vi "FPGAmain_utan_output.vi"() -> ()   [LabVIEW 2013]
uses:
  FPGA/DataMode.ctl
  FPGA/AcquireState.ctl
  FPGA/Input_5782/5782_states.ctl
  <vilib>/Platform/TimedLoop/XDataNode/timing_clust.ctl
  <vilib>/Platform/TimedLoop/XDataNode/nitl_modes.ctl
  <vilib>/Platform/TimedLoop/XDataNode/wakeup.ctl
  <vilib>/rvi/Emulation/niFpgaSctlEmulationGetInTimedLoop.vi
  <vilib>/rvi/Emulation/niFpgaEmulationReportErrorSimple.vi
  <vilib>/rvi/Emulation/niFpgaGetClockAttributes.vi
  <vilib>/rvi/eio/common/nirviEmuTemplateMethod_errors.vi
  <vilib>/rvi/Emulation/niFpgaCriticalErrorInLSC.vi
  <vilib>/rvi/FIFO/Fifo_Resource/nirvififoEmulationWriteFpgaImpl.vi
  <vilib>/rvi/DataTransferAndStorage/Container/Common/niFpgaContainerGetUniqueNameForEmu.vi
  <vilib>/rvi/FIFO/Fifo_Resource/nirvififoEmulationReadFpgaImpl.vi
  <vilib>/rvi/DataTransferAndStorage/Register/Emulation/niFpgaRegisterEmulationFpgaImpl.vi
  <instcachedir>/0/niFpgaRegisterEmulationFpgaImpl_DCF4BC0110594B98B44A971D60CEEC4D.lvgen/niFpgaRegisterEmulationFpgaImpl_DCF4BC0110594B98B44A971D60CEEC4D_016.vi
  <instcachedir>/0/niFpgaRegisterEmulationFpgaImpl_DCF4BC0110594B98B44A971D60CEEC4D.lvgen/niFpgaRegisterEmulationFpgaImpl_DCF4BC0110594B98B44A971D60CEEC4D_003.vi
  <instcachedir>/0/niFpgaRegisterEmulationFpgaImpl_DCF4BC0110594B98B44A971D60CEEC4D.lvgen/niFpgaRegisterEmulationFpgaImpl_DCF4BC0110594B98B44A971D60CEEC4D_014.vi
  <instcachedir>/0/niFpgaRegisterEmulationFpgaImpl_DCF4BC0110594B98B44A971D60CEEC4D.lvgen/niFpgaRegisterEmulationFpgaImpl_DCF4BC0110594B98B44A971D60CEEC4D_015.vi
  <vilib>/rvi/interface/RandomDataEmulation/nirviRandomDataMultiElementFPGAFIFO.vi
  <instcachedir>/0/nirviRandomDataMultiElementFPGAFIFO_F2B80EDE0D7944A08478D8D26097D4DB.lvgen/nirviRandomDataMultiElementFPGAFIFO_F2B80EDE0D7944A08478D8D26097D4DB_005.vi
  <vilib>/rvi/interface/RandomDataEmulation/niFpgaRandomDataHandleErrors.vi
  <vilib>/rvi/interface/RandomDataEmulation/nirviRandomDataFPGAFIFO.vi
  <instcachedir>/0/niFpgaRegisterEmulationFpgaImpl_DCF4BC0110594B98B44A971D60CEEC4D.lvgen/niFpgaRegisterEmulationFpgaImpl_DCF4BC0110594B98B44A971D60CEEC4D_009.vi
  <instcachedir>/0/niFpgaRegisterEmulationFpgaImpl_DCF4BC0110594B98B44A971D60CEEC4D.lvgen/niFpgaRegisterEmulationFpgaImpl_DCF4BC0110594B98B44A971D60CEEC4D_013.vi
  <vilib>/Platform/TimedLoop/XDataNode/XDataNode.xnode
  <vilib>/eio/EIONode/EIONode.xnode
  <vilib>/rvi/DataTransferAndStorage/Container/XNode/niFpgaContainer.xnode
  <vilib>/rvi/FIFO/Fifo_Resource/nirvififoEmulationWrite.vi
  <vilib>/rvi/FIFO/Fifo_Resource/nirvififoEmulationRead.vi
  <vilib>/rvi/DataTransferAndStorage/Register/Emulation/niFpgaRegisterEmulation.vi
  <vilib>/rvi/interface/RandomDataEmulation/nirviRandomDataFpgaMultiElementTemplate.vi
  <vilib>/rvi/interface/RandomDataEmulation/nirviRandomDataFpgaReadWriteTemplate.vi
  <vilib>/rvi/FIFO/Fifo_Resource/nirvififoEmulationP2P.vi
  <vilib>/Platform/TimedLoop/XDataNode/XDNodeRunTimeDep.lvlib
  <instrlib>/FlexRIO/Libraries/Helper VIs/NI FlexRIO Helper VIs.lvlib
panel:
  in  "delay phase":fxp<+,64,64>
  in  "AM phase":fxp<+,64,64>
  in  "Phase 5782":fxp<+,64,64>[](array[numeric])=[0.0, 0.0]
  in  "User Command Commit":bool
  in  "User Command":u8
  out "User Command Idle":bool
  out "User Command Status":u8
  in  "User Data 0":u8
  in  "User Data 1":u8
  out "PLL Locked":bool
  out "User Error":bool
  out "Configured?":bool
  in  "FIR coeffs":fxp<+/-,18,18>[](array[numeric])
  in  "Phase output":fxp<+,64,64>[](array[numeric])=[0.0, 0.0, 0.0, 0.0]
  in  "5782 record length":u16=4000 caption="Samples Per Trigger" min=1 step=1
  in  "Trigger Acquisition":bool
  in  "Continuous":bool
  out "IO Module\\Trigger Input":bool
  in  "Mode":T1
  in  "Simulated phase 5782":fxp<+,64,64>[](array[numeric])=[0.0, 0.0]
  in  "Acquisition running":bool
  in  "Samples Per Trigger":i32 min=1 step=1
  in  "Trigger simulated data":bool
  in  "simulated phase 5160":fxp<+,64,64>
  in  "phase 5160":fxp<+,64,64>
  # "Dynamic filter"
  # "Dynamic downsample"
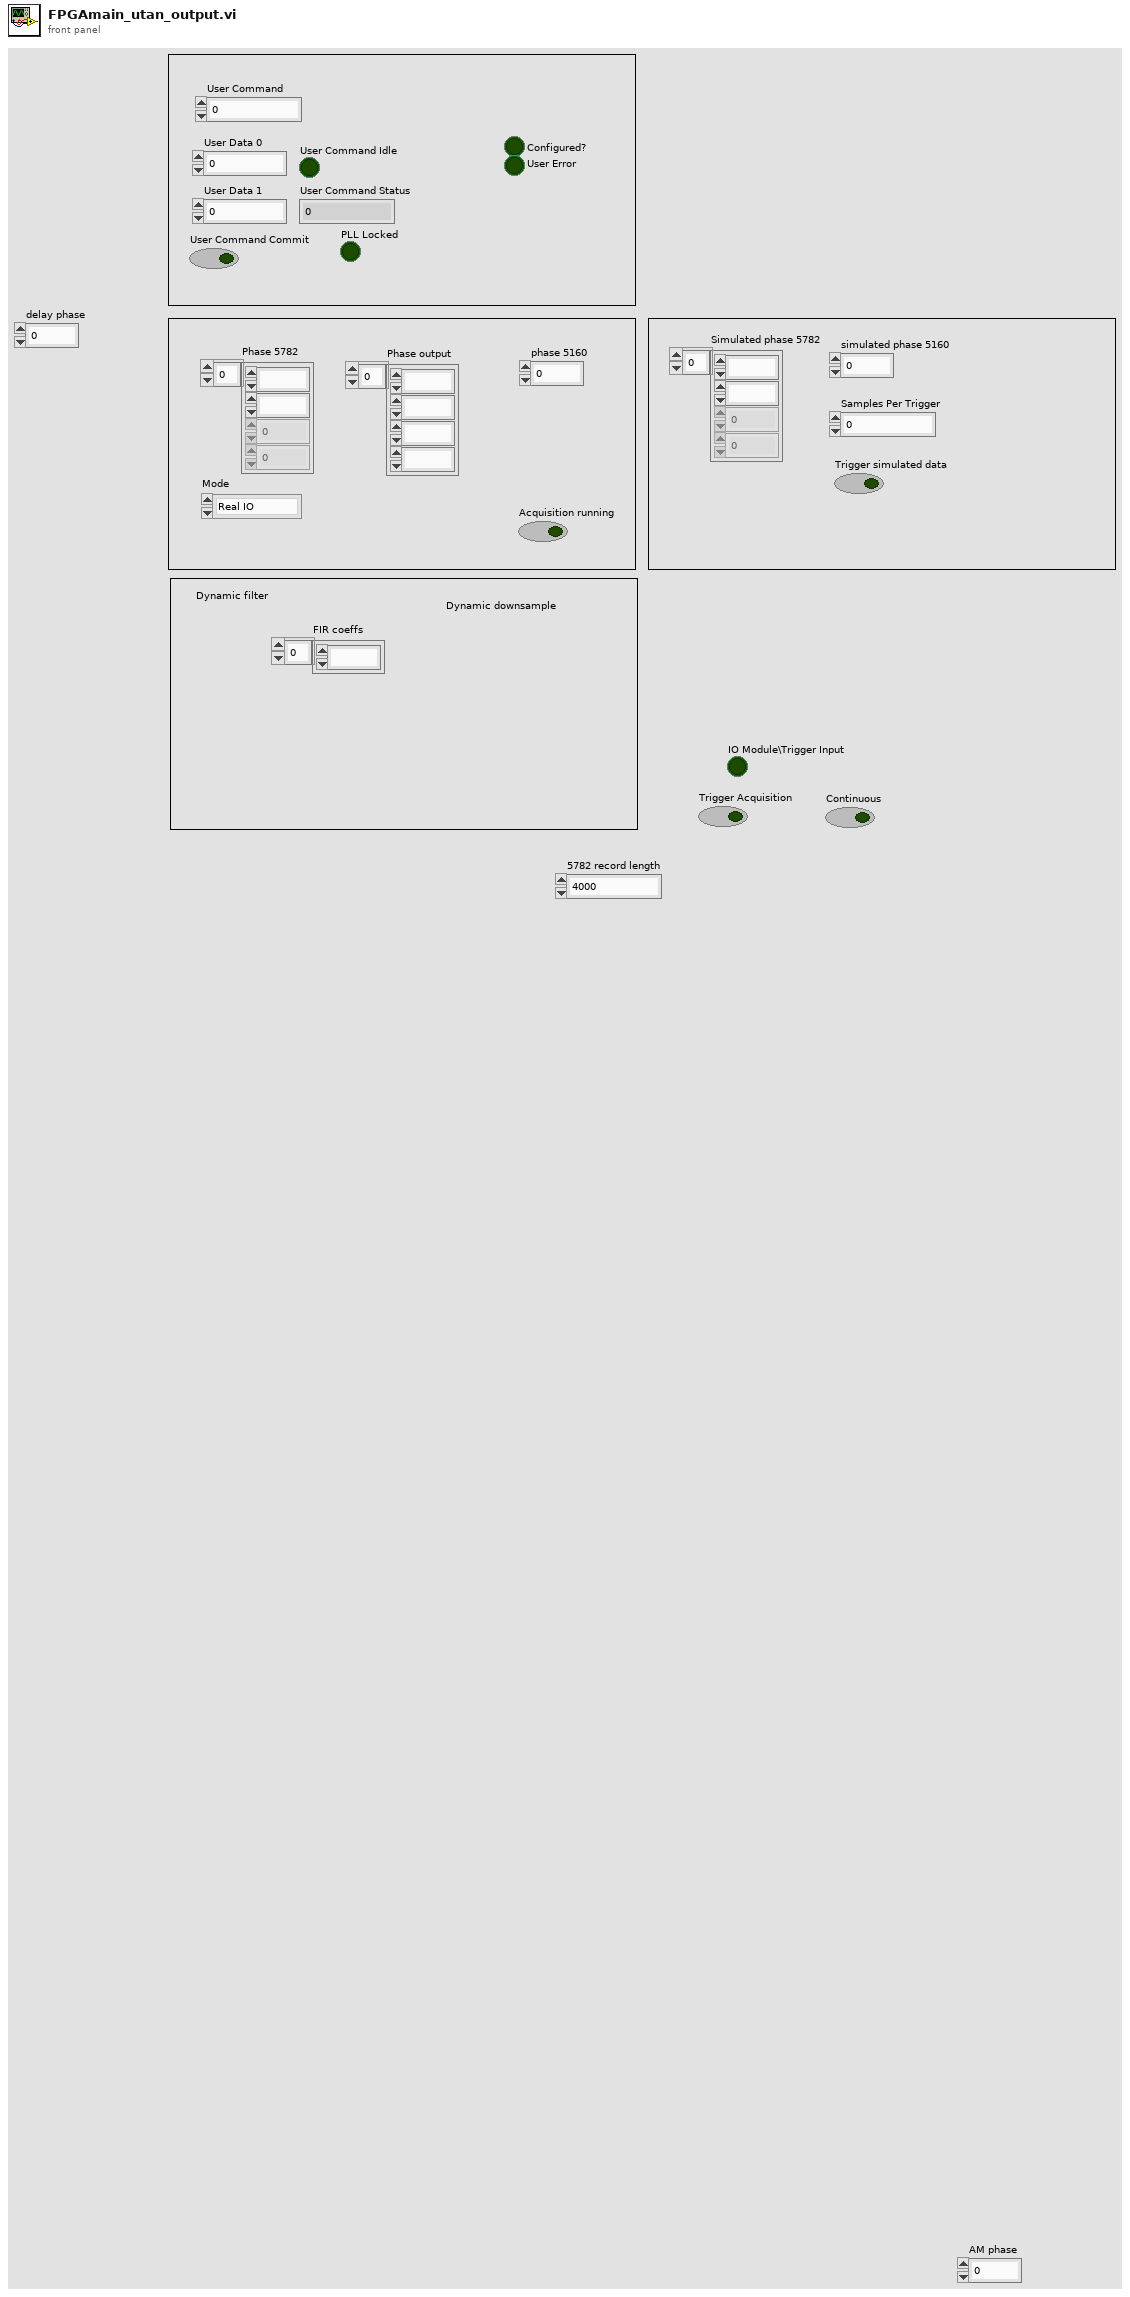
[diagram p1: front panel]
types:
  T1 = typedef "DataMode.ctl" = enum16{"Real IO", "Simulated"}
  T2 = typedef "5782_states.ctl" = enum8{"Wait for trigger", "Acquisition", "Send record length", "Quiet period"}
  T3 = typedef "AcquireState.ctl" = enum8{"Idle", "Acquire"}
  T4 = typedef "XDNodeRunTimeDep.lvlib/timing_clust.ctl" = cluster{"Expected End [f-1]":u64, "Actual End [f-1]":u64, "Finished Late? [f-1]":bool, "Expected End [i-1]":u64, "Actual End [i-1]":u64, "Finished Late? [i-1]":bool, "Expected Start [i]":u64, "Actual Start [i]":u64, "Expected Start [f]":u64, "Actual Start [f]":u64, "Source Name":string, "Structure Name":string, "Period":i64, "Deadline":i64, "Offset":i64, "Start":i64, "Priority":i32, "Timeout":i32, "Mode":T5, "Wakeup Reason":T6, "Error":errorcluster, "Source Type":string, "Secondary Source Type":string, "Global End Time":u64, "Global Start Time":u64, "Frame Duration":u64, "Iteration Duration":u64, "Assigned CPU":i32, "I/O Scan Engine Mode":u32}
  T5 = typedef "XDNodeRunTimeDep.lvlib/nitl_modes.ctl" = enum32{"No Change", "Process missed periods, maintain original phase", "Discard missed periods, maintain original phase", "Process missed periods, ignore original phase", "Discard missed periods, ignore original phase"}
  T6 = typedef "XDNodeRunTimeDep.lvlib/wakeup.ctl" = enum32{"Normal", "Aborted", "Asynchronous wakeup", "Timing source error", "Timed loop error", "Timeout"}
  T7 = typedef "I16 array size 2.ctl" = i16[]
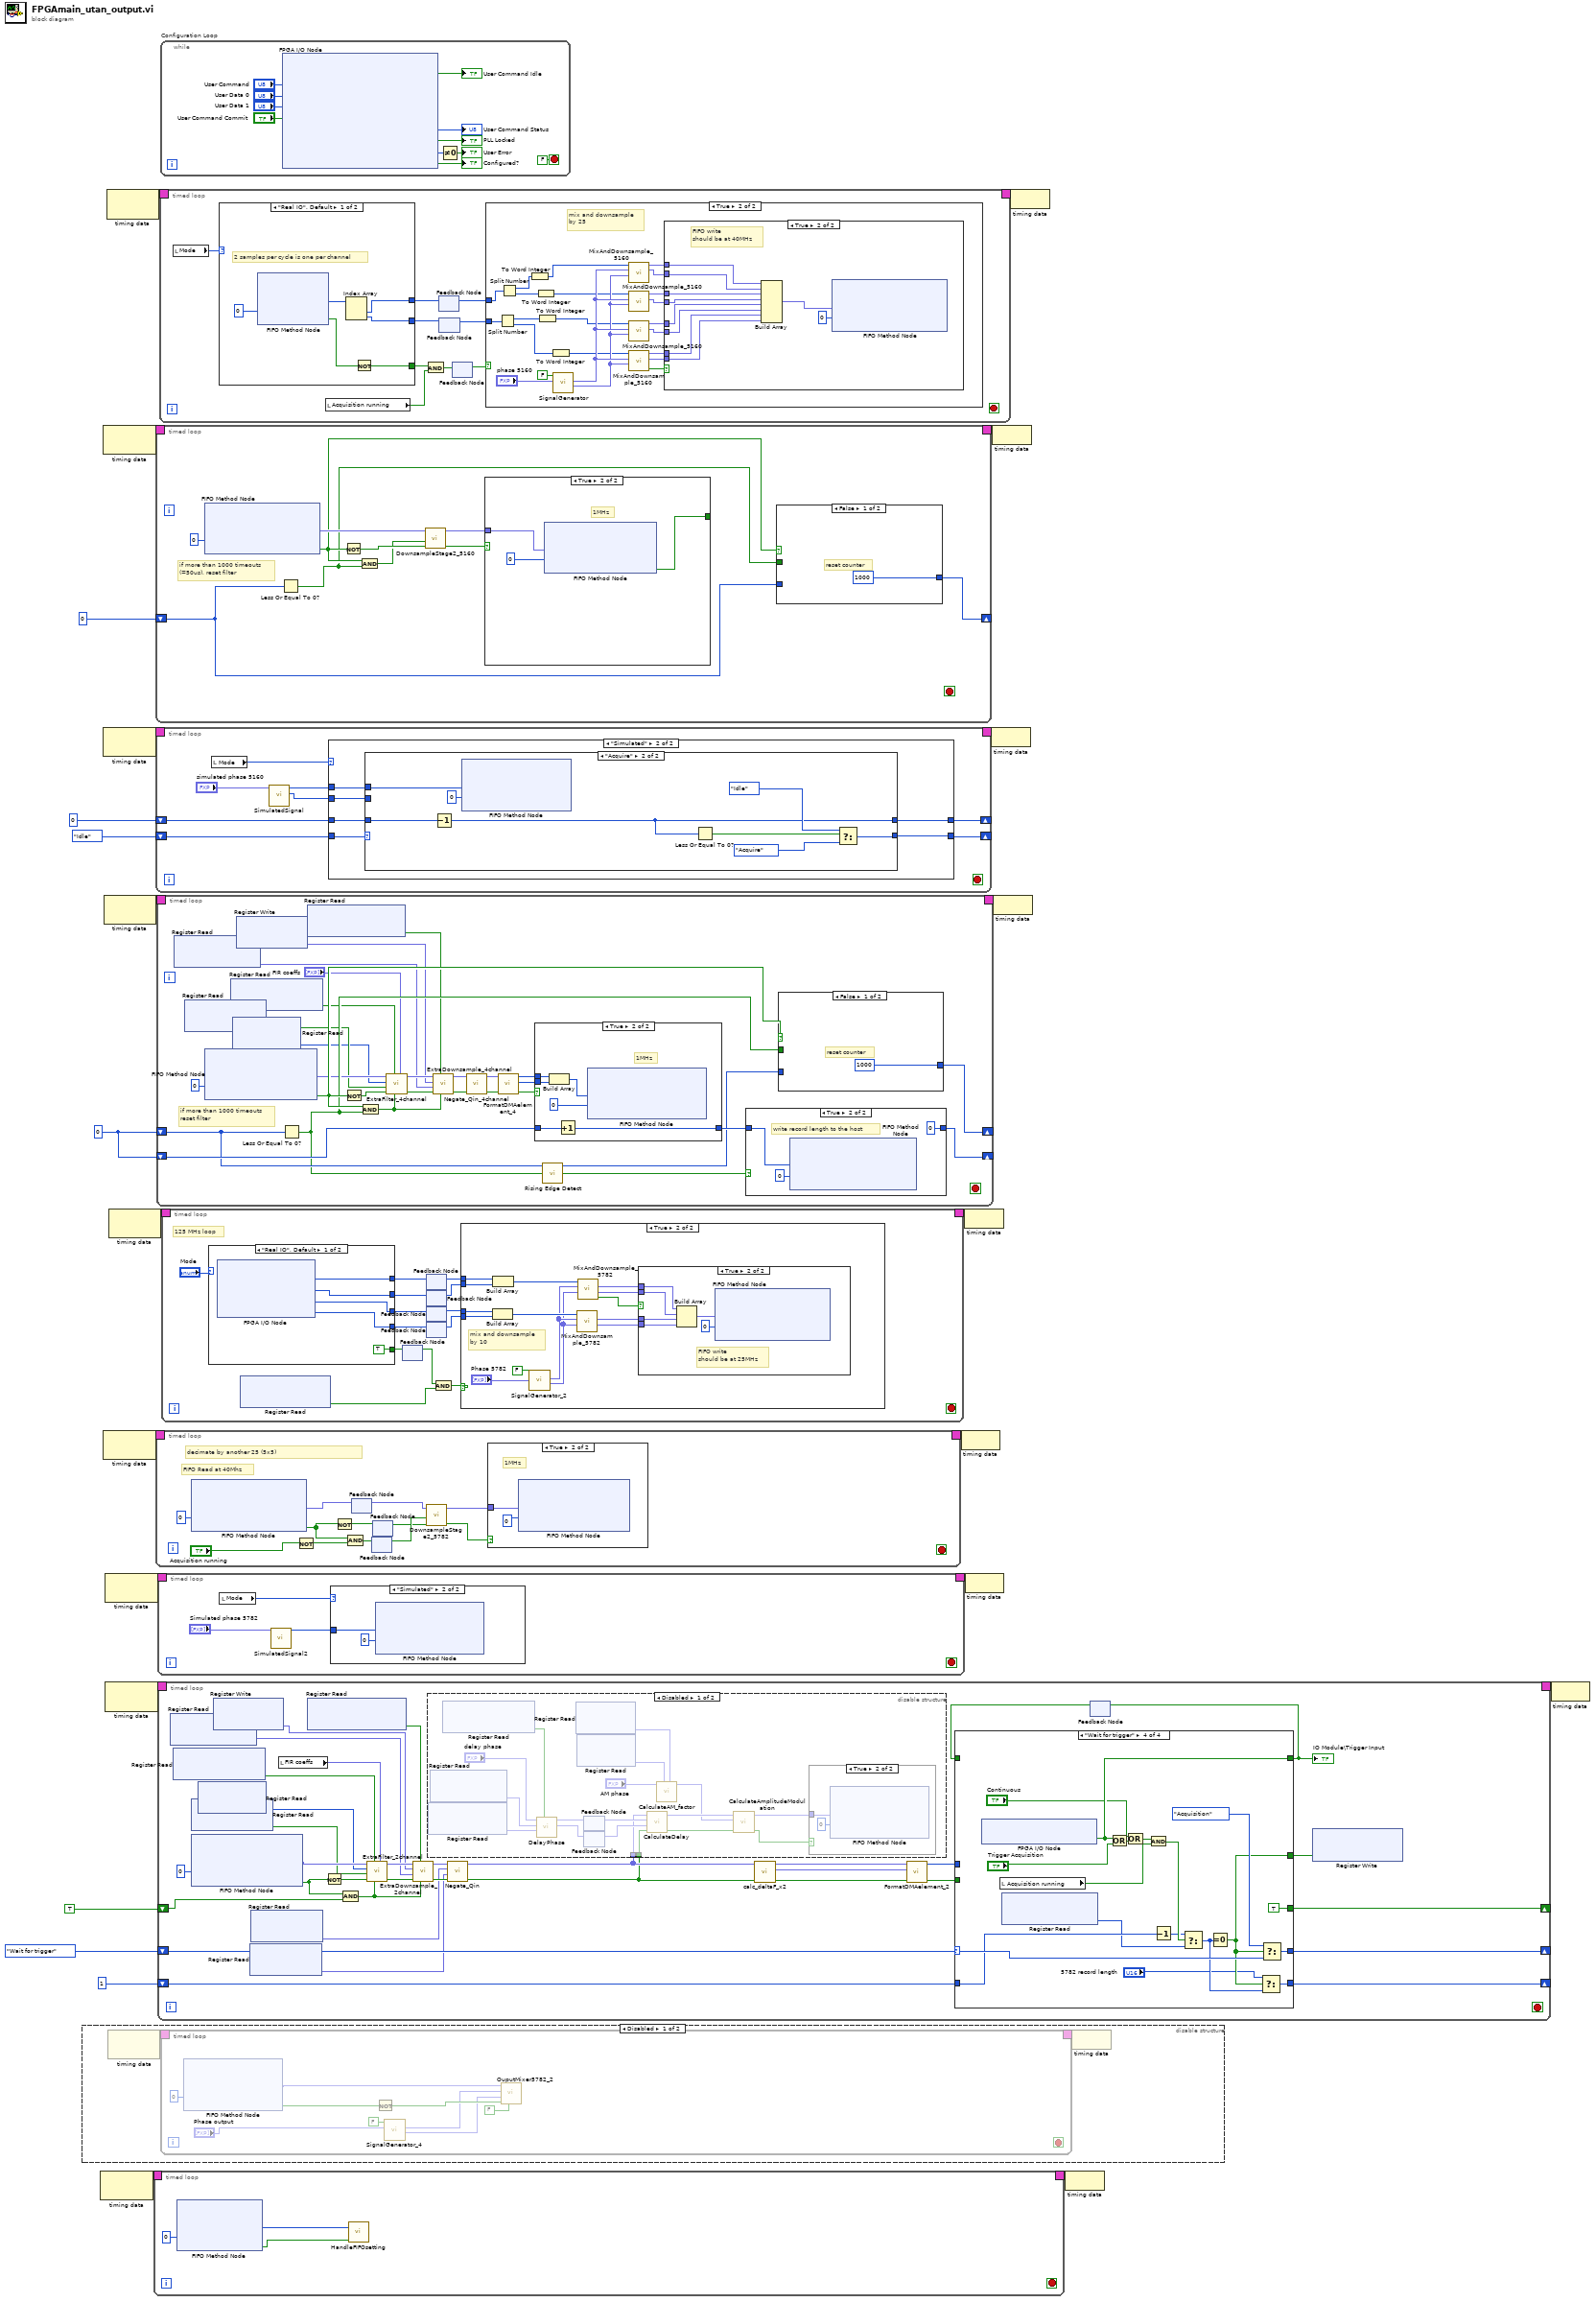
[diagram p0: block diagram]
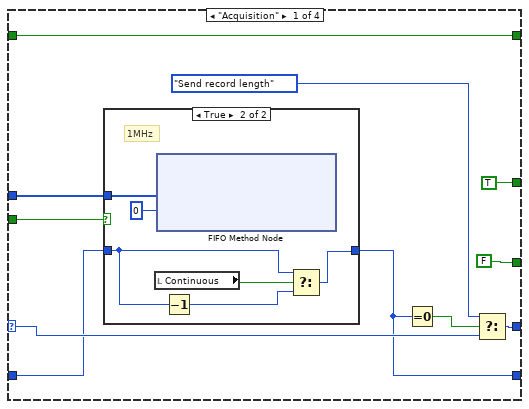
[diagram p5: hidden frame]
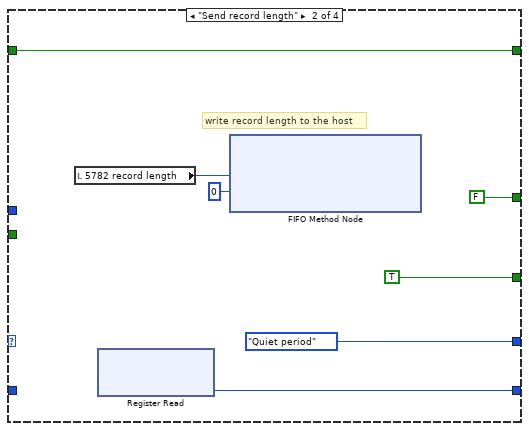
[diagram p7: hidden frame]
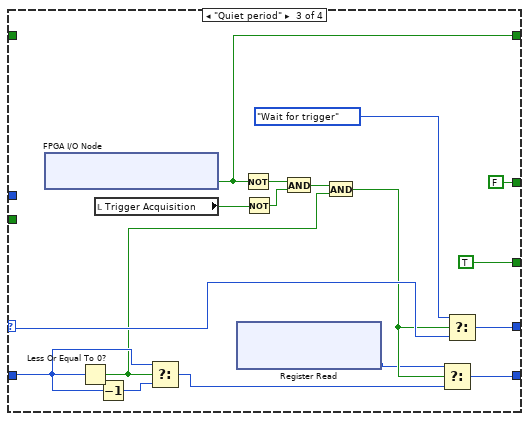
[diagram p8: hidden frame]
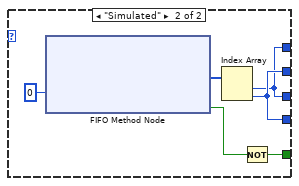
[diagram p11: hidden frame]
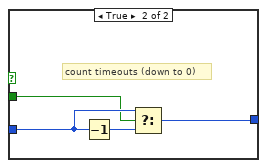
[diagram p14: hidden frame]
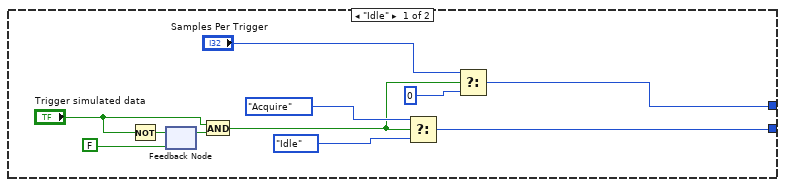
[diagram p18: hidden frame]
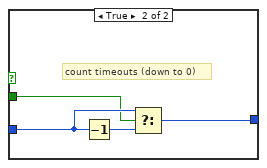
[diagram p19: hidden frame]
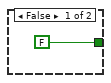
[diagram p20: hidden frame]
diagram:
  w14 = 0 ("y")
  n1 = disable-structure shown="Disabled" {
    frame Disabled {
      n2 = node-c288() -> (w27:T4)  [unwired: 1 in]
      n3 = timed-loop {
        timing: w27 -> [_]
        timing-out: [_] -> w26
        stop <- _ stop-if-true
        n4 = xnode ("FIFO Method Node")("Timeout"=0) -> ("Element"=w28:fxp<+/-,16,14>[], "Timed Out?"=w30:bool)  [unwired: 1 in, 1 out]
        n5 = Not(x=w30) -> (.not. x?=w34:bool)
        n6 = call "SignalGenerator_4.vi"("Phase"="Phase output", "reset"=FALSE) -> ("Sine out"=w31:fxp<+/-,16,0>[], "Cosine out"=w32:fxp<+/-,16,0>[])  [unwired: 8 in]
        n7 = call "OuputMixer5782_2.vi"("reset"=FALSE, "valid in"=w34, "Sine in"=w31, "Cosine in"=w32, "Data in"=w28) -> ()  [unwired: 5 in, 2 out]
      }
      n8 = node-c288(w26) -> ()
    }
    frame Enabled {
    }
  }
  n9 = node-c288() -> (w5:T4)  [unwired: 1 in]
  n10 = node-c288() -> (w23:T4)  [unwired: 1 in]
  n11 = node-c288() -> (w21:T4)  [unwired: 1 in]
  n12 = node-c288() -> (w11:T4)  [unwired: 1 in]
  n13 = node-c288() -> (w16:T4)  [unwired: 1 in]
  n14 = node-c288() -> (w13:T4)  [unwired: 1 in]
  n15 = node-c288() -> (w7:T4)  [unwired: 1 in]
  n16 = node-c288() -> (w25:T4)  [unwired: 1 in]
  n17 = node-c288() -> (w9:T4)  [unwired: 1 in]
  n18 = timed-loop {
    timing: w5 -> [_]
    timing-out: [_] -> w4
    stop <- _ stop-if-true
    n19 = xnode ("FIFO Method Node")("Timeout"=0) -> ("Element"=w42:u64, "Timed Out?"=w41:bool)  [unwired: 1 in, 1 out]
    n20 = call "HandleFIFOsetting.vi"("timed out"=w41, "Value"=w42) -> ()  [unwired: 10 in]
  }
  n21 = timed-loop {
    timing: w23 -> [_]
    timing-out: [_] -> w22
    shift-right: [w48] -> _
    shift-left: 0 ("y") -> [w47]
    stop <- _ stop-if-true
    # "if more than 1000 timeouts\n(=50us), reset filter"
    n22 = xnode ("FIFO Method Node")("Timeout"=0) -> ("Element"=w52:fxp<+/-,16,14>[], "Timed Out?"=w49:bool)  [unwired: 1 in, 1 out]
    n23 = Less Or Equal To 0?(x=w47) -> (x <= 0?=w46:bool)
    n24 = Not(x=w49) -> (.not. x?=w53:bool)
    n25 = And(x=w49, y=w46) -> (x .and. y?=w50:bool)
    n26 = call "DownsampleStage2_5160.vi"("valid in"=w53, "reset"=w50, "Element"=w52) -> ("valid out"=w54:bool, "Array"=w55:fxp<+/-,16,14>[])  [unwired: 7 in]
    n27 = case shown="True" w54 {
      tunnel: w55 -> [_ w62]
      tunnel: [FALSE ("Timed Out?") w63] -> _
      frame False {
      }
      frame True {
        # "1MHz"
        n28 = xnode ("FIFO Method Node")("Element"=w62, "Timeout"=0) -> ("Timed Out?"=w63:bool)  [unwired: 1 in, 1 out]
      }
    }
    n29 = case shown="False" w49 {
      tunnel: w46 -> [_ w58]
      tunnel: w47 -> [_ w59]
      tunnel: [1000 ("y") w57] -> w48
      frame False {
        # "reset counter"
      }
      frame True {
        # "count timeouts (down to 0)"
        n30 = Decrement(x=w59) -> (x-1=w60:i32)
        n31 = Select(t=w59, s=w58, f=w60) -> (s? t:f=w57:i32)
      }
    }
  }
  n32 = timed-loop {
    timing: w21 -> [_]
    timing-out: [_] -> w20
    shift-right: [w70] -> _
    shift-left: 0 ("f") -> [w69]
    shift-right: [w68] -> _
    shift-left: AcquireState."Idle" ("Acquire State") -> [w67]
    stop <- _ stop-if-true
    n33 = local read "Mode"() -> (w74:T1)
    n34 = call "SimulatedSignal.vi"("phase"="simulated phase 5160") -> ("cos output"=w72:i16, "Sample output"=w73:i16)  [unwired: 9 in]
    n35 = case shown="\"Simulated\"" w74 {
      tunnel: w73 -> [_ w82]
      tunnel: w72 -> [_ w77]
      tunnel: [w76 w81] -> w70
      tunnel: w69 -> [w76 w80]
      tunnel: [w75 w79] -> w68
      tunnel: w67 -> [w75 w78]
      frame "Real IO" {
      }
      frame "Simulated" {
        n36 = case shown="\"Acquire\"" w78 {
          tunnel: w80 -> [_ w98]
          tunnel: [w87 w97] -> w79
          tunnel: [w84 w96] -> w81
          tunnel: w82 -> [_ w95]
          tunnel: w77 -> [_ _]
          frame "Idle" {
            n37 = Not(x="Trigger simulated data") -> (.not. x?=w88:bool)
            n38 = feedback #1(FALSE) -> (w89:bool)
            n39 = feedback-in #1(w88) -> ()
            n40 = And(x="Trigger simulated data", y=w89) -> (x .and. y?=w83:bool)
            n41 = Select(t=AcquireState."Acquire" ("Acquire State"), s=w83, f=AcquireState."Idle" ("Acquire State")) -> (s? t:f=w87:T3)
            n42 = Select(t="Samples Per Trigger", s=w83, f=0) -> (s? t:f=w84:i32)
          }
          frame "Acquire" {
            n43 = Decrement(x=w98) -> (x-1=w96:i32)
            n44 = xnode ("FIFO Method Node")("Element"=w95, "Timeout"=0) -> ()  [unwired: 1 in, 2 out]
            n45 = Less Or Equal To 0?(x=w96) -> (x <= 0?=w100:bool)
            n46 = Select(t=AcquireState."Idle" ("Acquire State"), s=w100, f=AcquireState."Acquire" ("Acquire State")) -> (s? t:f=w97:T3)
          }
        }
      }
    }
  }
  n47 = timed-loop {
    timing: w11 -> [_]
    timing-out: [_] -> w10
    stop <- _ stop-if-true
    # "FIFO Read at 40Mhz"
    # "decimate by another 25 (5x5)"
    n48 = xnode ("FIFO Method Node")("Timeout"=0) -> ("Element"=w110:fxp<+/-,16,14>[], "Timed Out?"=w111:bool)  [unwired: 1 in, 1 out]
    n49 = Not(x="Acquisition running") -> (.not. x?=w112:bool)
    n50 = Not(x=w111) -> (.not. x?=w106:bool)
    n51 = And(x=w111, y=w112) -> (x .and. y?=w108:bool)
    n52 = feedback #2() -> (w109:fxp<+/-,16,14>[])  [unwired: 1 in]
    n53 = feedback-in #2(w110) -> ()
    n54 = feedback #3() -> (w107:bool)  [unwired: 1 in]
    n55 = feedback-in #3(w108) -> ()
    n56 = feedback #4() -> (w105:bool)  [unwired: 1 in]
    n57 = feedback-in #4(w106) -> ()
    n58 = call "DownsampleStage2_5782.vi"("valid in"=w105, "reset"=w107, "Data in"=w109) -> ("valid out"=w113:bool, "data out"=w114:fxp<+/-,16,14>[])  [unwired: 7 in]
    n59 = case shown="True" w113 {
      tunnel: w114 -> [_ w116]
      frame False {
      }
      frame True {
        # "1MHz"
        n60 = xnode ("FIFO Method Node")("Element"=w116, "Timeout"=0) -> ()  [unwired: 1 in, 2 out]
      }
    }
  }
  n61 = timed-loop {
    timing: w16 -> [_]
    timing-out: [_] -> w15
    shift-right: [w142] -> _
    shift-left: w14 -> [w141]
    shift-right: [w144] -> _
    shift-left: w14 -> [w146]
    stop <- _ stop-if-true
    # "if more than 1000 timeouts\nreset filter"
    n62 = xnode ("Register Read")() -> ("Data"=w123:fxp<+,8,8>)  [unwired: 1 in, 1 out]
    n63 = xnode ("Register Read")() -> ("Data"=w121:bool)  [unwired: 1 in, 1 out]
    n64 = xnode ("FIFO Method Node")("Timeout"=0) -> ("Element"=w137:fxp<+/-,16,14>[], "Timed Out?"=w143:bool)  [unwired: 1 in, 1 out]
    n65 = xnode ("Register Read")() -> ("Data"=w122:bool)  [unwired: 1 in, 1 out]
    n66 = xnode ("Register Read")() -> ("Data"=w120:i32)  [unwired: 1 in, 1 out]
    n67 = xnode ("Register Write")() -> ("Data"=w124:fxp<+/-,32,1>)  [unwired: 1 in, 1 out]
    n68 = Less Or Equal To 0?(x=w141) -> (x <= 0?=w140:bool)
    n69 = xnode ("Register Read")() -> ("Data"=w125:bool)  [unwired: 1 in, 1 out]
    n70 = Not(x=w143) -> (.not. x?=w136:bool)
    n71 = And(x=w143, y=w140) -> (x .and. y?=w138:bool)
    n72 = call "ExtraFilter_4channel.vi"(5:"new coeffs"="FIR coeffs", "reset"=w138, 7:"new coeffs"=w122, "valid in"=w136, "enable filter"=w121, "new shift"=w120, "Data in"=w137) -> ("valid out"=w127:bool, "Data out"=w128:fxp<+/-,16,14>[])  [unwired: 3 in]
    n73 = call "ExtraDownsample_4channel.vi"("reset"=w138, "Set downsample"=w125, "valid in"=w127, "Downsample"=w123, "CIC Gain"=w124, "Data in"=w128) -> ("valid out"=w129:bool, "Data out"=w132:fxp<+/-,16,14>[])  [unwired: 4 in]
    n74 = call "Negate_Qin_4channel.vi"("valid in"=w129, "Data in"=w132) -> ("valid out"=w130:bool, "Data out"=w131:fxp<+/-,16,14>[])  [unwired: 8 in]
    n75 = call "FormatDMAelement_4.vi"("valid in"=w130, "Data in"=w131) -> ("valid out"=w133:bool, "Element2"=w134:u64, "Element1"=w135:u64)  [unwired: 7 in]
    n76 = case shown="True" w133 {
      tunnel: w135 -> [_ w162]
      tunnel: w134 -> [_ w161]
      tunnel: w146 -> [w157 w159]
      tunnel: [w157 w158] -> w145
      frame False {
      }
      frame True {
        # "1MHz"
        n77 = Build Array(w162, w161) -> (w160:u64[])
        n78 = Increment(x=w159) -> (x+1=w158:i32)
        n79 = xnode ("FIFO Method Node")("Element"=w160, "Timeout"=0) -> ()  [unwired: 1 in, 2 out]
      }
    }
    n80 = call <instrlib>:"Rising Edge Detect.vi"("signal"=w140) -> ("edge detected"=w139:bool)  [unwired: 14 in]
    n81 = case shown="True" w139 {
      tunnel: w145 -> [w153 w154]
      tunnel: [w153 0 ("y")] -> w144
      frame False {
      }
      frame True {
        # "write record length to the host"
        n82 = xnode ("FIFO Method Node")("Element"=w154, "Timeout"=0) -> ()  [unwired: 1 in, 2 out]
      }
    }
    n83 = case shown="False" w143 {
      tunnel: w140 -> [_ w150]
      tunnel: w141 -> [_ w151]
      tunnel: [1000 ("y") w149] -> w142
      frame False {
        # "reset counter"
      }
      frame True {
        # "count timeouts (down to 0)"
        n84 = Decrement(x=w151) -> (x-1=w152:i32)
        n85 = Select(t=w151, s=w150, f=w152) -> (s? t:f=w149:i32)
      }
    }
  }
  n86 = timed-loop {
    timing: w13 -> [_]
    timing-out: [_] -> w12
    stop <- _ stop-if-true
    n87 = local read "Mode"() -> (w168:T1)
    n88 = call "SimulatedSignal2.vi"("Phase"="Simulated phase 5782") -> ("output"=w167:T7)  [unwired: 9 in, 1 out]
    n89 = case shown="\"Simulated\"" w168 {
      tunnel: w167 -> [_ w169]
      frame "Real IO", Default {
      }
      frame "Simulated" {
        n90 = xnode ("FIFO Method Node")("Element"=w169, "Timeout"=0) -> ()  [unwired: 1 in, 2 out]
      }
    }
  }
  n91 = timed-loop {
    timing: w7 -> [_]
    timing-out: [_] -> w6
    shift-right: [w204] -> _
    shift-left: 5782_states."Wait for trigger" ("5782 states") -> [w206]
    shift-right: [w203] -> _
    shift-left: u16 1 ("trigger samples") -> [w205]
    shift-right: [w192] -> _
    shift-left: TRUE -> [w195]
    stop <- _ stop-if-true
    n92 = xnode ("Register Read")() -> ("Data"=w177:fxp<+,8,8>)  [unwired: 1 in, 1 out]
    n93 = xnode ("Register Read")() -> ("Data"=w183:bool)  [unwired: 1 in, 1 out]
    n94 = xnode ("Register Read")() -> ("Data"=w178:bool)  [unwired: 1 in, 1 out]
    n95 = xnode ("FIFO Method Node")("Timeout"=0) -> ("Element"=w197:fxp<+/-,16,14>[], "Timed Out?"=w196:bool)  [unwired: 1 in, 1 out]
    n96 = xnode ("Register Read")() -> ("Data"=w179:i32)  [unwired: 1 in, 1 out]
    n97 = xnode ("Register Write")() -> ("Data"=w176:fxp<+/-,32,1>)  [unwired: 1 in, 1 out]
    n98 = xnode ("Register Read")() -> ("Data"=w181:fxp<+/-,16,14>)  [unwired: 1 in, 1 out]
    n99 = xnode ("Register Read")() -> ("Data"=w182:fxp<+/-,16,14>)  [unwired: 1 in, 1 out]
    n100 = local read "FIR coeffs"() -> (w175:fxp<+/-,18,18>[])
    n101 = xnode ("Register Read")() -> ("Data"=w180:bool)  [unwired: 1 in, 1 out]
    n102 = Not(x=w196) -> (.not. x?=w199:bool)
    n103 = And(x=w196, y=w195) -> (x .and. y?=w201:bool)
    n104 = call "ExtraFilter_2channel.vi"(5:"new coeffs"=w175, "reset"=w201, 7:"new coeffs"=w183, "valid in"=w199, "enable filter"=w178, "new shift"=w179, "Data in"=w197) -> ("valid out"=w200:bool, "Data out"=w198:fxp<+/-,16,14>[])  [unwired: 3 in]
    n105 = call "ExtraDownsample_2channel.vi"("reset"=w201, "Set downsample"=w180, "valid in"=w200, "Downsample"=w177, "CIC Gain"=w176, "Data in"=w198) -> ("valid out"=w189:bool, "Data out"=w190:fxp<+/-,16,14>[])  [unwired: 4 in]
    n106 = call "Negate_Qin.vi"("valid in"=w189, "DC offset chan 1"=w181, "DC offset chan 0"=w182, "Data in"=w190) -> ("valid out"=w186:bool, "Data out"=w188:fxp<+/-,16,14>[])  [unwired: 6 in]
    n107 = disable-structure shown="Disabled" {
      disable-tunnel: w188 -> [w217 _]
      disable-tunnel: w186 -> [w213 _]
      frame Disabled {
        n108 = xnode ("Register Read")() -> ("Data"=w208:fxp<+/-,16,0>)  [unwired: 1 in, 1 out]
        n109 = xnode ("Register Read")() -> ("Data"=w209:fxp<+/-,16,0>)  [unwired: 1 in, 1 out]
        n110 = xnode ("Register Read")() -> ("Data"=w210:bool)  [unwired: 1 in, 1 out]
        n111 = call "DelayPhase.vi"("Use fixed delay"=w210, "fixed cos_fi"=w208, "fixed sin fi"=w209, "delay phase"="delay phase") -> ("cos_fi"=w215:fxp<+/-,16,0>, "sin fi"=w216:fxp<+/-,16,0>)  [unwired: 6 in]
        n112 = xnode ("Register Read")() -> ("Data"=w212:fxp<+/-,16,2>)  [unwired: 1 in, 1 out]
        n113 = xnode ("Register Read")() -> ("Data"=w211:fxp<+/-,16,2>)  [unwired: 1 in, 1 out]
        n114 = feedback #5() -> (w224:fxp<+/-,16,0>)  [unwired: 1 in]
        n115 = feedback-in #5(w216) -> ()
        n116 = feedback #6() -> (w223:fxp<+/-,16,0>)  [unwired: 1 in]
        n117 = feedback-in #6(w215) -> ()
        n118 = call "CalculateDelay.vi"("input valid"=w213, "cos_fi"=w223, "sin fi"=w224, "Data in"=w217) -> ("output valid"=w221:bool, "Data out"=w222:fxp<+/-,16,14>[])  [unwired: 6 in]
        n119 = call "CalculateAM_factor.vi"("b_am"=w212, "a_am"=w211, "AM phase"="AM phase") -> ("AM_factor"=w218:fxp<+/-,16,2>)  [unwired: 7 in, 1 out]
        n120 = call "CalculateAmplitudeModulation.vi"("input valid"=w221, "AM_factor"=w218, "Data in"=w222) -> ("output valid"=w219:bool, "Data out"=w220:fxp<+/-,16,14>[])  [unwired: 7 in]
        n121 = case shown="True" w219 {
          tunnel: w220 -> [_ w225]
          frame False {
          }
          frame True {
            n122 = xnode ("FIFO Method Node")("Element"=w225, "Timeout"=0) -> ()  [unwired: 1 in, 2 out]
          }
        }
      }
      frame Enabled {
      }
    }
    n123 = call "calc_deltaF_x2.vi"("valid in"=w186, "Data in"=w188) -> ("valid out"=w185:bool, "deltaF"=w184:fxp<+/-,32,30>[], "Data out"=w187:fxp<+/-,16,14>[])  [unwired: 7 in]
    n124 = call "FormatDMAelement_2.vi"("valid in"=w185, "deltaF"=w184, "Data in"=w187) -> ("valid out"=w193:bool, "Element"=w194:u64[])  [unwired: 7 in]
    n125 = feedback #7() -> (w174:bool)  [unwired: 1 in]
    n126 = case shown="\"Wait for trigger\"" w206 {
      selector: w206 -> [w237 _ w267 w286]
      tunnel: w205 -> [w233 _ w255 w275]
      tunnel: [w236 5782_states."Quiet period" ("5782 states") w266 w285] -> w204
      tunnel: [w230 w245 w268 w284] -> w203
      tunnel: w194 -> [w231 _ _ _]
      tunnel: w193 -> [w232 _ _ _]
      tunnel: [FALSE TRUE TRUE TRUE] -> w192
      tunnel: [TRUE FALSE ("5782 triggered") FALSE ("5782 triggered") w279] -> w191
      tunnel: [w229 w246 w257 w278] -> w173
      tunnel: w174 -> [w229 w246 _ _]
      frame "Acquisition" {
        n127 = case shown="True" w232 {
          tunnel: w231 -> [_ w244]
          tunnel: [w238 w241] -> w230
          tunnel: w233 -> [w238 w239]
          frame False {
          }
          frame True {
            # "1MHz"
            n128 = local read "Continuous"() -> (w242:bool)
            n129 = xnode ("FIFO Method Node")("Element"=w244, "Timeout"=0) -> ()  [unwired: 1 in, 2 out]
            n130 = Decrement(x=w239) -> (x-1=w240:u16)
            n131 = Select(t=w239, s=w242, f=w240) -> (s? t:f=w241:u16)
          }
        }
        n132 = Equal To 0?(x=w230) -> (x = 0?=w234:bool)
        n133 = Select(t=5782_states."Send record length" ("5782 states"), s=w234, f=w237) -> (s? t:f=w236:T2)
      }
      frame "Send record length" {
        # "write record length to the host"
        n134 = local read "5782 record length"() -> (w248:u16)
        n135 = xnode ("Register Read")() -> ("Data"=w245:u16)  [unwired: 1 in, 1 out]
        n136 = xnode ("FIFO Method Node")("Element"=w248, "Timeout"=0) -> ()  [unwired: 1 in, 2 out]
      }
      frame "Quiet period" {
        n137 = xnode "FPGA I/O Node"() -> ("IO Module\\Trigger Input"=w257:bool)  [unwired: 1 in, 1 out]
        n138 = Less Or Equal To 0?(x=w255) -> (x <= 0?=w254:bool)
        n139 = local read "Trigger Acquisition"() -> (w263:bool)
        n140 = Decrement(x=w255) -> (x-1=w256:u16)
        n141 = Select(t=w255, s=w254, f=w256) -> (s? t:f=w253:u16)
        n142 = xnode ("Register Read")() -> ("Data"=w252:u16)  [unwired: 1 in, 1 out]
        n143 = Not(x=w257) -> (.not. x?=w262:bool)
        n144 = Not(x=w263) -> (.not. x?=w261:bool)
        n145 = And(x=w262, y=w261) -> (x .and. y?=w260:bool)
        n146 = And(x=w260, y=w254) -> (x .and. y?=w265:bool)
        n147 = Select(t=w252, s=w265, f=w253) -> (s? t:f=w268:u16)
        n148 = Select(t=5782_states."Wait for trigger" ("5782 states"), s=w265, f=w267) -> (s? t:f=w266:T2)
      }
      frame "Wait for trigger" {
        n149 = xnode "FPGA I/O Node"() -> ("IO Module\\Trigger Input"=w278:bool)  [unwired: 1 in, 1 out]
        n150 = local read "Acquisition running"() -> (w280:bool)
        n151 = xnode ("Register Read")() -> ("Data"=w272:u16)  [unwired: 1 in, 1 out]
        n152 = Or(x=w278, y="Trigger Acquisition") -> (x .or. y?=w274:bool)
        n153 = Or(x="Continuous", y=w274) -> (x .or. y?=w273:bool)
        n154 = And(x=w273, y=w280) -> (x .and. y?=w281:bool)
        n155 = Decrement(x=w275) -> (x-1=w276:u16)
        n156 = Select(t=w276, s=w281, f=w272) -> (s? t:f=w277:u16)
        n157 = Equal To 0?(x=w277) -> (x = 0?=w279:bool)
        n158 = Select(t="5782 record length", s=w279, f=w277) -> (s? t:f=w284:u16)
        n159 = Select(t=5782_states."Acquisition" ("5782 states"), s=w279, f=w286) -> (s? t:f=w285:T2)
      }
    }
    "IO Module\\Trigger Input" <- w173
    n160 = feedback-in #7(w173) -> ()
    n161 = xnode ("Register Write")("Data"=w191) -> ()  [unwired: 1 in, 1 out]
  }
  n162 = timed-loop {
    timing: w25 -> [_]
    timing-out: [_] -> w24
    stop <- _ stop-if-true
    n163 = local read "Mode"() -> (w292:T1)
    n164 = case shown="\"Real IO\", Default" w292 {
      tunnel: [w334 w340] -> w297
      tunnel: [w331 w337] -> w291
      tunnel: [w333 w340] -> w294
      frame "Real IO", Default {
        # "2 samples per cycle is one per channel"
        n165 = xnode ("FIFO Method Node")("Timeout"=0) -> ("Element"=w336:u32[], "Timed Out?"=w332:bool)  [unwired: 1 in, 1 out]
        n166 = Index Array(array=w336) -> (element #1=w334:u32, element #2=w333:u32)  [unwired: 2 in]
        n167 = Not(x=w332) -> (.not. x?=w331:bool)
      }
      frame "Simulated" {
        n168 = xnode ("FIFO Method Node")("Timeout"=0) -> ("Element"=w339:i16, "Timed Out?"=w338:bool)  [unwired: 1 in, 1 out]
        n169 = Not(x=w338) -> (.not. x?=w337:bool)
        n170 = Join Numbers(hi=w339, lo=w339) -> ((hi.lo)=w340:u32)
      }
    }
    n171 = local read "Acquisition running"() -> (w290:bool)
    n172 = And(x=w291, y=w290) -> (x .and. y?=w289:bool)
    n173 = feedback-in #8(w297) -> ()
    n174 = feedback #8() -> (w296:u32)  [unwired: 1 in]
    n175 = feedback #9() -> (w293:u32)  [unwired: 1 in]
    n176 = feedback-in #9(w294) -> ()
    n177 = feedback #10() -> (w295:bool)  [unwired: 1 in]
    n178 = feedback-in #10(w289) -> ()
    n179 = case shown="True" w295 {
      tunnel: w296 -> [_ w311]
      tunnel: w293 -> [_ w300]
      frame False {
        # "FIFO read timeout, no data"
      }
      frame True {
        # "mix and downsample\nby 25"
        n180 = Split Number(x=w300) -> (hi(x)=w301:u16, lo(x)=w302:u16)
        n181 = Split Number(x=w311) -> (hi(x)=w310:u16, lo(x)=w309:u16)
        n182 = To Word Integer(number=w310) -> (16bit integer=w304:i16)
        n183 = To Word Integer(number=w309) -> (16bit integer=w303:i16)
        n184 = To Word Integer(number=w301) -> (16bit integer=w298:i16)
        n185 = To Word Integer(number=w302) -> (16bit integer=w299:i16)
        n186 = call "SignalGenerator.vi"("phase"="phase 5160", "Reset"=FALSE) -> ("Cos"=w305:fxp<+/-,16,0>, "Sin"=w306:fxp<+/-,16,0>)  [unwired: 7 in, 1 out]
        n187 = call "MixAndDownsample_5160.vi"("Sine in"=w305, "Cosine in"=w306, "Sample in"=w304) -> ("Q out"=w318:fxp<+/-,16,14>, "I out"=w320:fxp<+/-,16,14>)  [unwired: 6 in, 1 out]
        n188 = call "MixAndDownsample_5160.vi"("Sine in"=w305, "Cosine in"=w306, "Sample in"=w303) -> ("Q out"=w316:fxp<+/-,16,14>, "I out"=w317:fxp<+/-,16,14>)  [unwired: 6 in, 1 out]
        n189 = call "MixAndDownsample_5160.vi"("Sine in"=w305, "Cosine in"=w306, "Sample in"=w298) -> ("Q out"=w314:fxp<+/-,16,14>, "I out"=w315:fxp<+/-,16,14>)  [unwired: 6 in, 1 out]
        n190 = call "MixAndDownsample_5160.vi"("Sine in"=w305, "Cosine in"=w306, "Sample in"=w299) -> ("valid out"=w319:bool, "Q out"=w312:fxp<+/-,16,14>, "I out"=w313:fxp<+/-,16,14>)  [unwired: 6 in]
        n191 = case shown="True" w319 {
          tunnel: w320 -> [_ w329]
          tunnel: w318 -> [_ w328]
          tunnel: w317 -> [_ w327]
          tunnel: w316 -> [_ w321]
          tunnel: w315 -> [_ w326]
          tunnel: w314 -> [_ w325]
          tunnel: w313 -> [_ w324]
          tunnel: w312 -> [_ w323]
          frame False {
          }
          frame True {
            # "FIFO write\nshould be at 40MHz"
            n192 = Build Array(w329, w328, w327, w321, w326, w325, w324, w323) -> (w322:fxp<+/-,16,14>[])
            n193 = xnode ("FIFO Method Node")("Element"=w322, "Timeout"=0) -> ()  [unwired: 1 in, 2 out]
          }
        }
      }
    }
  }
  n194 = while "Configuration Loop" {
    stop <- FALSE stop-if-true
    n195 = xnode "FPGA I/O Node"("IO Module\\User Command"="User Command", "IO Module\\User Data 0"="User Data 0", "IO Module\\User Data 1"="User Data 1", "IO Module\\User Command Commit"="User Command Commit") -> ("IO Module\\User Command Idle"=→"User Command Idle":bool, "IO Module\\User Command Status"=→"User Command Status":u8, "IO Module\\PLL Locked"=→"PLL Locked":bool, "IO Module\\User Error"=w349:u8, "IO Module\\Initialization Done"=→"Configured?":bool)  [unwired: 9 in, 9 out]
    n196 = Not Equal To 0?(x=w349) -> (x != 0?=→"User Error":bool)
  }
  n197 = timed-loop {
    timing: w9 -> [_]
    timing-out: [_] -> w8
    stop <- _ stop-if-true
    # "125 MHz loop"
    n198 = case shown="\"Real IO\", Default" "Mode" {
      tunnel: [w393 w396] -> w366
      tunnel: [w392 w397] -> w364
      tunnel: [w391 w396] -> w362
      tunnel: [w390 w397] -> w359
      tunnel: [TRUE w394] -> w358
      frame "Real IO", Default {
        n199 = xnode "FPGA I/O Node"() -> ("IO Module\\AI 0 N-1"=w393:i16, "IO Module\\AI 0 N"=w392:i16, "IO Module\\AI 1 N-1"=w391:i16, "IO Module\\AI 1 N"=w390:i16)  [unwired: 4 in, 4 out]
      }
      frame "Simulated" {
        n200 = xnode ("FIFO Method Node")("Timeout"=0) -> ("Element"=w398:i16[], "Timed Out?"=w395:bool)  [unwired: 1 in, 1 out]
        n201 = Index Array(array=w398) -> (element #1=w396:i16, element #2=w397:i16)  [unwired: 2 in]
        n202 = Not(x=w395) -> (.not. x?=w394:bool)
      }
    }
    n203 = xnode ("Register Read")() -> ("Data"=w356:bool)  [unwired: 1 in, 1 out]
    n204 = feedback #11() -> (w357:bool)  [unwired: 1 in]
    n205 = feedback-in #11(w358) -> ()
    n206 = feedback #12() -> (w365:i16)  [unwired: 1 in]
    n207 = feedback-in #12(w366) -> ()
    n208 = feedback #13() -> (w363:i16)  [unwired: 1 in]
    n209 = feedback-in #13(w364) -> ()
    n210 = feedback #14() -> (w361:i16)  [unwired: 1 in]
    n211 = feedback-in #14(w362) -> ()
    n212 = feedback #15() -> (w360:i16)  [unwired: 1 in]
    n213 = feedback-in #15(w359) -> ()
    n214 = And(x=w357, y=w356) -> (x .and. y?=w367:bool)
    n215 = case shown="True" w367 {
      tunnel: w365 -> [_ w373]
      tunnel: w363 -> [_ w372]
      tunnel: w361 -> [_ w371]
      tunnel: w360 -> [_ w370]
      frame False {
      }
      frame True {
        # "mix and downsample\nby 10"
        n216 = Build Array(w371, w370) -> (w382:i16[])
        n217 = Build Array(w373, w372) -> (w369:i16[])
        n218 = call "SignalGenerator_2.vi"("Phase"="Phase 5782", "reset"=FALSE) -> ("Sine out"=w374:fxp<+/-,16,0>[], "Cosine out"=w375:fxp<+/-,16,0>[])  [unwired: 8 in]
        n219 = call "MixAndDownsample_5782.vi"("Sine in"=w374, "Cosine in"=w375, "Signal Input"=w382) -> ("Q out"=w377:fxp<+/-,16,14>, "I out"=w378:fxp<+/-,16,14>)  [unwired: 6 in, 1 out]
        n220 = call "MixAndDownsample_5782.vi"("Sine in"=w374, "Cosine in"=w375, "Signal Input"=w369) -> ("data valid"=w379:bool, "Q out"=w380:fxp<+/-,16,14>, "I out"=w381:fxp<+/-,16,14>)  [unwired: 6 in]
        n221 = case shown="True" w379 {
          tunnel: w380 -> [_ w388]
          tunnel: w381 -> [_ w385]
          tunnel: w378 -> [_ w384]
          tunnel: w377 -> [_ w383]
          frame False {
          }
          frame True {
            # "FIFO write\nshould be at 25MHz"
            n222 = Build Array(w385, w388, w384, w383) -> (w387:fxp<+/-,16,14>[])
            n223 = xnode ("FIFO Method Node")("Element"=w387, "Timeout"=0) -> ()  [unwired: 1 in, 2 out]
          }
        }
      }
    }
  }
  n224 = node-c288(w10) -> ()
  n225 = node-c288(w8) -> ()
  n226 = node-c288(w12) -> ()
  n227 = node-c288(w20) -> ()
  n228 = node-c288(w22) -> ()
  n229 = node-c288(w15) -> ()
  n230 = node-c288(w24) -> ()
  n231 = node-c288(w4) -> ()
  n232 = node-c288(w6) -> ()
